vi "format console (SubVI).vi"(9 "Caption.Text":string, 11 "String ref in":refnum<vi>) -> (3 "String ref out":refnum<vi>)   [LabVIEW 2021]
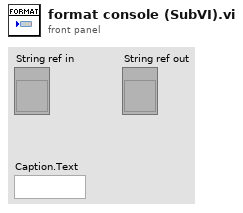
[diagram p1: front panel]
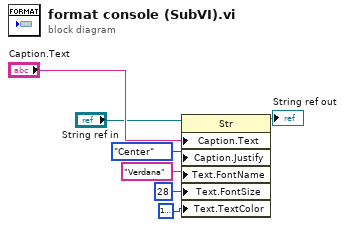
[diagram p0: block diagram]
diagram:
  n1 = property class="Str"(reference="String ref in", "Caption.Text"="Caption.Text", "Caption.Justify"=enum16{"Left", "Center", "Right"}."Center" ("Caption.Justification"), "Text.FontName"="Verdana" ("Text.Font:Name"), "Text.FontSize"=u32 28 ("Text.Font:Size"), "Text.TextColor"=u32 16777228 ("Text.Text Colors:Text Color")) -> (reference out=→"String ref out":refnum<vi>)  [unwired: 1 in, 1 out]
